vi "create_plot_line.vi"(6 "plot ID":i32, 7 "color vector":dbl[](array[numeric]), 8 "z vector":dbl[](array[numeric]), 9 "y vector":dbl[](array[numeric]), 10 "x vector":dbl[](array[numeric]), 11 "plots in":refnum<class "Base Datatype.lvclass">[](array[class])) -> (3 "plots out":refnum<class "Base Datatype.lvclass">[](array[class]))   [LabVIEW 2020, in "3DPC_SurfacePlot.xctl"]
doc: "Plots a line or curve in terms of x, y, and z points. This VI has three 1D array inputs that specify each point on the line or curve."
uses:
  <vilib>/Native 3D Graph/xcontrol/3DPC_SurfacePlot.xctl
  <vilib>/Native 3D Graph/classes/Base Datatype.lvclass
  <vilib>/Native 3D Graph/classes/Line/Line.lvclass
  e:/builds/penguin/labview/branches/2020/dev/dist/vi.lib/Native 3D Graph/classes/Base Datatype.lvclass
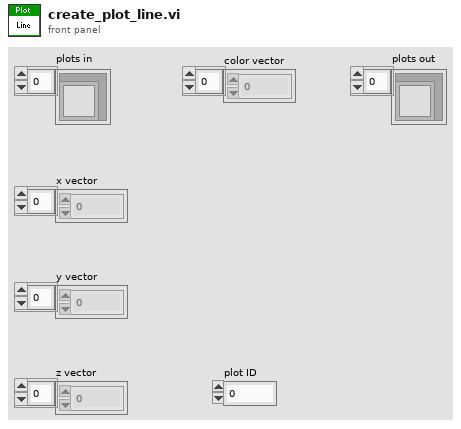
[diagram p1: front panel]
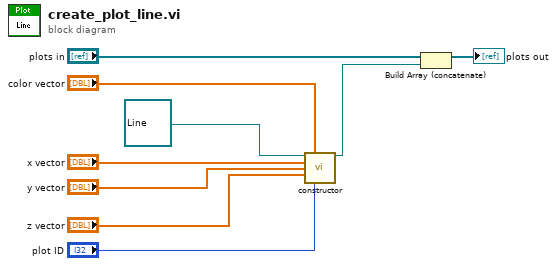
[diagram p0: block diagram]
diagram:
  n1 = call-dynamic "constructor.vi"("Line in"=refnum<class "Line.lvclass"> refnum ("Surface in"), "Color Vector"="color vector", "X Vector"="x vector", "Y Vector"="y vector", "Z Vector"="z vector", "Plot ID"="plot ID") -> ("Line out"=w5:refnum<class "Line.lvclass">)  [unwired: 1 in, 8 out]
  n2 = Build Array (concatenate)("plots in", w5) -> (→"plots out":refnum<class "Base Datatype.lvclass">[])
